vi "AlliGator Convert Phasor Plot Point to Phasor.vi"(9 "Phasor Plot Reference Points":T3, 11 "Phasor Plot Point":T2) -> (3 "Phasor":T1)   [LabVIEW 2021, in "AlliGator Phasor Plot.lvlib"]
doc: "Converts Phasor Plot image coordinates to actual phasor value."
uses:
  AlliGator Phasor Plot.lvlib
  Phasor Ratio/AlliGator Phasor Plot Reference Points.ctl
  Image/Image Point.ctl
  Phasor/Phasor (g, s).ctl
  Phasor/Phasor.lvlib
  Phasor Ratio/AlliGator Phasor Ratio.lvlib
  Image/Image.lvlib
panel:
  # "see the AlliGator License on the block diagram (Ctrl+E or Window:Show Block Diagram)"
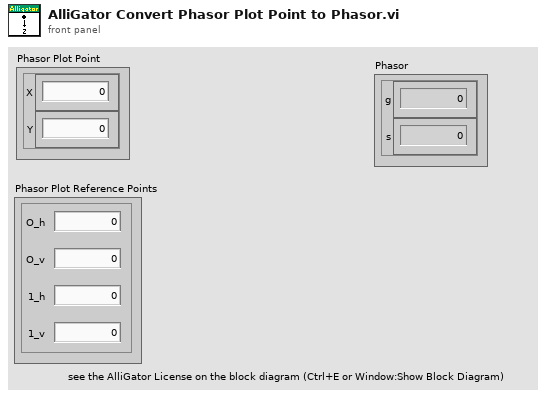
[diagram p1: front panel]
types:
  T1 = typedef "Phasor.lvlib/Phasor (g, s).ctl" = cluster{"g":dbl, "s":dbl}
  T2 = typedef "Image.lvlib/Image Point.ctl" = cluster{"X":i32, "Y":i32}
  T3 = typedef "AlliGator Phasor Ratio.lvlib/AlliGator Phasor Plot Reference Points.ctl" = cluster{"O_h":dbl, "O_v":dbl, "1_h":dbl, "1_v":dbl}
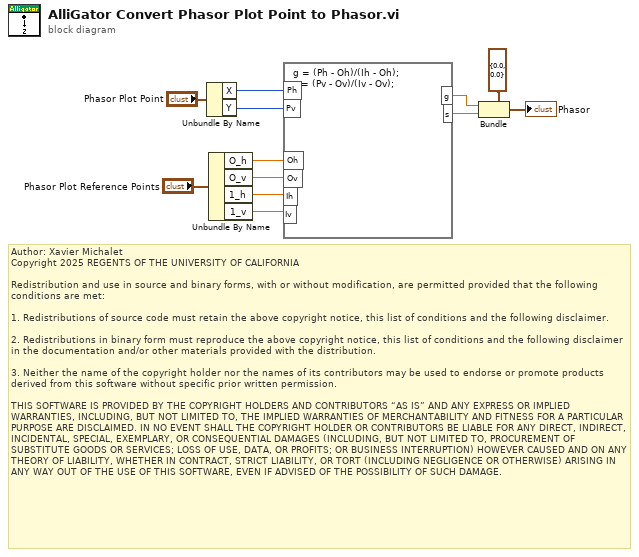
[diagram p0: block diagram]
diagram:
  # "Author: Xavier Michalet\nCopyright 2025 REGENTS OF THE UNIVERSITY OF CALIFORNIA\n\nRedistribution and use in source and binary forms, with or without modification, are permitted provided that the following conditions are met:\n\n1. Redistributions of source code must retain the above copyright notice, this list of conditions and the following disclaimer.\n\n2. Redistributions in binary form must reproduce the above copyright notice, this list of conditions and the following disclaimer in the documentation and/or other materials provided with the distribution.\n\n3. Neither the name of the copyright holder nor the names of its contributors may be used to endorse or promote products derived from this software without specific prior written permission.\n\nTHIS SOFTWARE IS PROVIDED BY THE COPYRIGHT HOLDERS AND CONTRIBUTORS “AS IS” AND ANY EXPRESS OR IMPLIED WARRANTIES, INCLUDING, BUT NOT LIMITED TO, THE IMPLIED WARRANTIES OF MERCHANTABILITY AND FITNESS FOR A PARTICULAR PURPOSE ARE DISCLAIMED. IN NO EVENT SHALL THE COPYRIGHT HOLDER OR CONTRIBUTORS BE LIABLE FOR ANY DIRECT, INDIRECT, INCIDENTAL, SPECIAL, EXEMPLARY, OR CONSEQUENTIAL DAMAGES (INCLUDING, BUT NOT LIMITED TO, PROCUREMENT OF SUBSTITUTE GOODS OR SERVICES; LOSS OF USE, DATA, OR PROFITS; OR BUSINESS INTERRUPTION) HOWEVER CAUSED AND ON ANY THEORY OF LIABILITY, WHETHER IN CONTRACT, STRICT LIABILITY, OR TORT (INCLUDING NEGLIGENCE OR OTHERWISE) ARISING IN ANY WAY OUT OF THE USE OF THIS SOFTWARE, EVEN IF ADVISED OF THE POSSIBILITY OF SUCH DAMAGE."
  n1 = Unbundle By Name("Phasor Plot Point") -> ("X"=w10:i32, "Y"=w9:i32)
  n2 = Unbundle By Name("Phasor Plot Reference Points") -> ("O_h"=w8:dbl, "O_v"=w7:dbl, "1_h"=w6:dbl, "1_v"=w5:dbl)
  n3 = formula code="g = (Ph - Oh)/(Ih - Oh);\ns = (Pv - Ov)/(Iv - Ov);"("Ph"=w10, "Pv"=w9, "Oh"=w8, "Ov"=w7, "Ih"=w6, "Iv"=w5) -> ("g"=w3:dbl, "s"=w2:dbl)
  n4 = Bundle(cluster=T1 {"g"=0.0, "s"=0.0} ("Phasor"), "g"=w3, "s"=w2) -> (→"Phasor":T1)
